vi "SDI-12 Single Calibration output cluster.vi"(0 "RS232 Port In":refnum<visa-resource-name>="COM11", 1 "Sensor Address In":string="0", 3 "Cumulative Volume":dbl, 7 "Error In (No Error)":errorcluster, 12 "Time Array In":dbl[](array[numeric]), 13 "Measurement Array In":dbl[][](array[numeric])) -> (14 "time array out":dbl[](array[numeric]), 15 "Measurements Out":dbl[](array[numeric]), 17 "Array":timestamp[](array[timestamp]), 21 "Address Out":string="a" caption="sensor address out", 22 "Measurement  array Out":dbl[][](array[numeric]), 23 "output cluster":T1 caption="Cluster" {"Salinity" format="%_3g"; "Temp\ndeg C" format="%_2g"; "ORP" format="%_4g"; "pH" format="%_4g"; "Dissolved\nOxygen mg/L" format="%_3g"; "Specific\nCond (mS)" format="%_4g"; "Cumulative\nVolume (ml)" format="%#_4g"}, 24 "Temperature":cluster{"Y":dbl[], "Y":dbl[]}[](graph), 25 "Sonde Data Display":T2, 27 "Error Out":errorcluster)   [LabVIEW 2016]
doc: "A general set of examples of the SDI-12 API for a generic sensor. A tab control separates each example, and contains the following examples:\n1. Read Single.\n2. Read Multiple.\n3. Acknowledge Active.\n4. Change Address.\n5. Address Query.\n6. Send Identification."
uses:
  SDI-12/Sonde Vertical Graph.ctl
  Waterloo DAQ/controls/Vertical Chart.ctl
  activeXtest/activeXtest 2015 Folder/sonde cluster.ctl
  SDI-12/SDI-12.lvlib
panel:
  out "loop counter":i32
  out "Error Out 3":errorcluster
  out "error out 2":errorcluster
  out "Error Out 2":errorcluster
  out "Sensor On/Off Response":bool
  out "Battery Voltage (V)":dbl
  out "Number of Measurements Out":i32
  in  "Measurement Type In (Normal)":i32(ring)=1 items=["Normal", "Concurrent", "Continuous"]
  out "Parameter Out":i32(ring) items=["0", "1", "2", "3", "4", "5", "6", "7", "8", "9"]
  in  "Parameter In (0)":i32(ring) items=["0", "1", "2", "3", "4", "5", "6", "7", "8", "9"]
  in  "CRC (False)":bool
  out "CRC Out":bool
  out "Measurement Type Out":i32(ring) items=["Normal", "Concurrent", "Continuous"]
  out "Time (s)":dbl
  out "start time":timestamp
  # "deg C"
  # "pH"
  # "specific conductance"
  # "salinity"
  # "DO % saturation"
  # "DO mg/L"
  # "ORP"
  # "depth"
  # "battery"
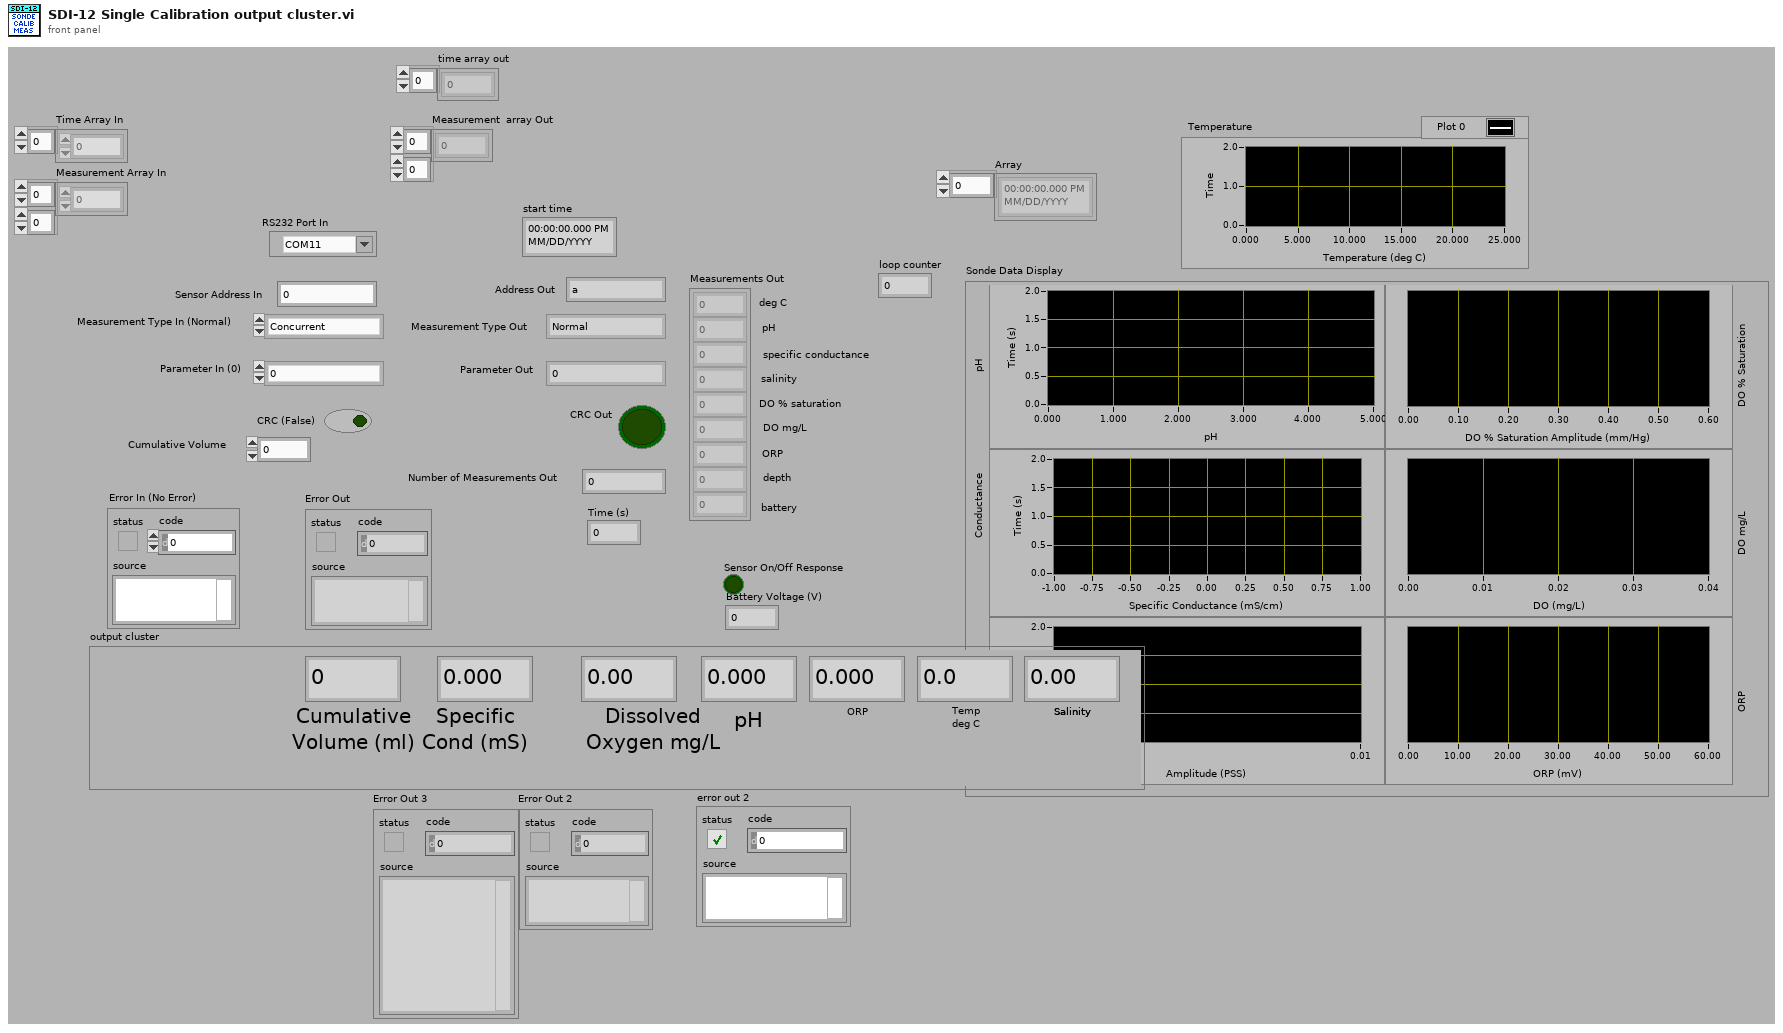
[diagram p1: front panel]
types:
  T1 = typedef "sonde cluster.ctl" = cluster{"Cumulative\nVolume (ml)":dbl, "Specific\nCond (mS)":dbl, "Dissolved\nOxygen mg/L":dbl, "pH":dbl, "ORP":dbl, "Temp\ndeg C":dbl, "Salinity":dbl}
  T2 = typedef "Sonde Vertical Graph.ctl" = cluster{"pH":T3, "Conductance":T3, "Salinity":T3, "DO % Saturation":T3, "DO mg/L":T3, "ORP":T3}
  T3 = typedef "Vertical Chart.ctl" = cluster{"Y":dbl[], "Y":dbl[]}[]
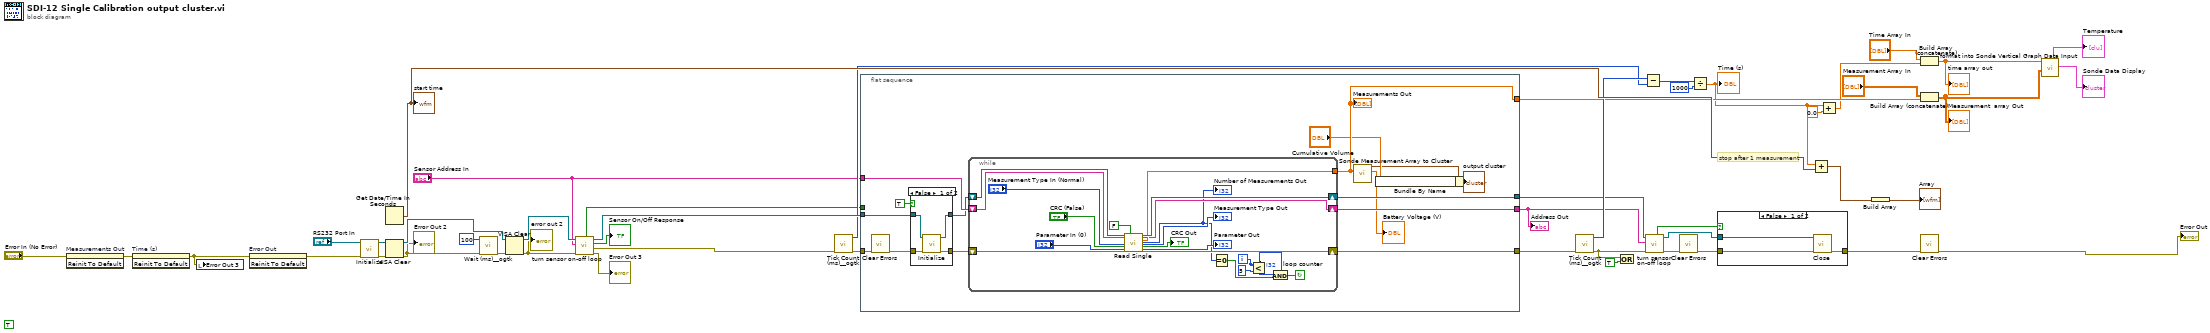
[diagram p0: block diagram]
diagram:
  (unwired) TRUE ("Sensor On/Off")
  # "stop after 1 measurement"
  n1 = invoke on="Measurements Out" class="Arr (strict)" method="Reinit To Default"(error in="Error In (No Error)") -> (error out=w4:errorcluster)  [unwired: 2 in, 2 out]
  n2 = invoke on="Time (s)" class="DigNum (strict)" method="Reinit To Default"(error in=w4) -> (error out=w2:errorcluster)  [unwired: 2 in, 2 out]
  n3 = local write "Error Out 3"(w2) -> ()
  n4 = invoke on="Error Out" class="Clust (strict)" method="Reinit To Default"(error in=w2) -> (error out=w23:errorcluster)  [unwired: 2 in, 2 out]
  n5 = call "Initialize.vi"("Error In (No Error)"=w23, "RS232 Port In"="RS232 Port In") -> ("Error Out"=w15:errorcluster, "RS232 Port Out"=w47:refnum<visa-resource-name>)  [unwired: 8 in]
  n6 = Get Date/Time In Seconds() -> (seconds since 1Jan1904=w42:timestamp)
  "start time" <- w42
  n7 = VISA Clear(VISA resource name=w47, error in (no error)=w15) -> (VISA resource name out=w16:refnum<visa-resource-name>, error out=w14:errorcluster)
  "Error Out 2" <- w14
  n8 = call "Wait (ms)__ogtk.vi"("error in (no error)"=w14, "milliseconds to wait"=u32 100) -> ("error out"=w20:errorcluster)  [unwired: 8 in, 1 out]
  n9 = VISA Clear(VISA resource name=w16, error in (no error)=w20) -> (VISA resource name out=w22:refnum<visa-resource-name>, error out=w21:errorcluster)
  "error out 2" <- w21
  n10 = call "turn sensor on-off loop.vi"("error in (no error)"=w21, "Address Out"="Sensor Address In", "VISA Refnum in"=w22) -> ("error out"=→"Error Out 3":errorcluster, "error out 2"=w38:errorcluster, "Sensor On/Off Response"=→"Sensor On/Off Response":bool, "VISA Refnum out"=w37:refnum<visa-resource-name>, "Initialize/Close?"=w13:bool)  [unwired: 4 in]
  n11 = call "Tick Count (ms)__ogtk.vi"("error in (no error)"=w38) -> ("error out"=w35:errorcluster, "millisecond timer value"=w33:u32)  [unwired: 9 in]
  n12 = flat-sequence {
    tunnel: [w63] -> w10
    tunnel: [w62] -> w36
    tunnel: w35 -> [w61]
    tunnel: w37 -> [w53]
    tunnel: [w59] -> w30
    tunnel: "Sensor Address In" -> [w60]
    tunnel: [w58] -> w7
    tunnel: w13 -> [_]
    frame #0 {
      n13 = call <vilib>:"Clear Errors.vi"("error in (no error)"=w61) -> ("error out"=w54:errorcluster)  [unwired: 5 in, 1 out]
      n14 = case shown="False" TRUE {
        tunnel: w54 -> [w87 w89]
        tunnel: w53 -> [w86 w88]
        tunnel: [w85 w89] -> w52
        tunnel: [w84 w88] -> w51
        frame False {
          n15 = call "Initialize.vi"("Error In (No Error)"=w87, "RS232 Port In"=w86) -> ("Error Out"=w85:errorcluster, "RS232 Port Out"=w84:refnum<visa-resource-name>)  [unwired: 8 in]
        }
        frame True {
        }
      }
      n16 = while {
        tunnel: [w74] -> w59
        shift-right: [w73] -> w58
        shift-left: w60 -> [w75]
        shift-right: [w82] -> w62
        shift-left: w52 -> [w72]
        shift-right: [w83] -> w63
        shift-left: w51 -> [w71]
        i -> [w66]
        stop <- w67 continue-if-true
        n17 = call "Read Single.vi"("RS232 Port In"=w71, "Sensor Address In"=w75, "Measurement Type In (Normal)"="Measurement Type In (Normal)", "CRC (False)"="CRC (False)", "Parameter In (0)"="Parameter In (0)", "Error In (No Error)"=w72, "Initialize/close"=FALSE) -> ("RS232 Port Out"=w83:refnum<visa-resource-name>, "Sensor Address Out"=w73:string, "Measurements Out"=w74:dbl[], "Number of Measurements Out"=w69:i32, "Measurement Type Out"=→"Measurement Type Out":i32, "CRC Out"=→"CRC Out":bool, "Parameter Out"=→"Parameter Out":i32, "Error Out"=w82:errorcluster)  [unwired: 13 in]
        "Number of Measurements Out" <- w69
        n18 = Equal To 0?(x=w69) -> (x = 0?=w68:bool)
        n19 = Less?(x=w66, y=5) -> (x < y?=w64:bool)
        n20 = And(x=w64, y=w68) -> (x .and. y?=w67:bool)
        "loop counter" <- w66
      }
      "Measurements Out" <- w59
      n21 = call "Sonde Measurement Array to Cluster.vi"("Measurements In"=w59) -> ("Battery Voltage (V)"=→"Battery Voltage (V)":dbl, "Sonde Data Cluster"=w56:T1)  [unwired: 9 in]
      n22 = Bundle By Name(cluster=w56, "Cumulative\nVolume (ml)"="Cumulative Volume") -> (→"output cluster":T1)
    }
  }
  n23 = call "Tick Count (ms)__ogtk.vi"("error in (no error)"=w36) -> ("error out"=w9:errorcluster, "millisecond timer value"=w34:u32)  [unwired: 9 in]
  n24 = Compound Arithmetic op=OR(w9, TRUE) -> ()  [unwired: 1 out]
  n25 = Subtract(x=w34, y=w33) -> (x-y=w32:u32)
  n26 = call "turn sensor on-off loop.vi"("error in (no error)"=w9, "Address Out"=w7, "VISA Refnum in"=w10) -> ("error out"=w6:errorcluster, "VISA Refnum out"=w8:refnum<visa-resource-name>, "Initialize/Close?"=w5:bool)  [unwired: 4 in, 2 out]
  n27 = call <vilib>:"Clear Errors.vi"("error in (no error)"=w6) -> ("error out"=w17:errorcluster)  [unwired: 5 in, 1 out]
  n28 = Divide(x=w32, y=u32 1000) -> (x/y=w29:dbl)
  "Time (s)" <- w29
  n29 = case shown="False" w5 {
    tunnel: [w92 w93] -> w43
    tunnel: w17 -> [w91 w93]
    tunnel: w8 -> [w90 _]
    frame False {
      n30 = call "Close.vi"("Error In (No Error)"=w91, "RS232 Port In"=w90) -> ("Error Out"=w92:errorcluster)  [unwired: 9 in]
    }
    frame True {
    }
  }
  n31 = Add(x=w29, y=w42) -> (x+y=w45:timestamp)
  n32 = Add(x=w29, y=0.0) -> (x+y=w28:dbl)
  n33 = Build Array(w45) -> (→"Array":timestamp[])
  n34 = Build Array (concatenate)("Time Array In", w28) -> (w40:dbl[])
  "time array out" <- w40
  n35 = Build Array (concatenate)("Measurement Array In", w30) -> (w44:dbl[][])
  "Measurement  array Out" <- w44
  n36 = call <vilib>:"Clear Errors.vi"("error in (no error)"=w43) -> ("error out"=→"Error Out":errorcluster)  [unwired: 5 in, 1 out]
  n37 = call "format into Sonde Vertical Graph Data Input.vi"("Sonde Measurement Array"=w44, "Time Array"=w40) -> ("Sonde Data Display"=→"Sonde Data Display":T2, "Temperature"=→"Temperature":cluster{"X":dbl[], "Y":dbl[]}[])  [unwired: 8 in]
  "Address Out" <- w7
